vi "Allocate Memory.vi"(4 "Type":variant, 5 "error in (no error)":errorcluster, 8 "Size":i32) -> (0 "Error out":errorcluster, 3 "Data Pointer":i32)   [LabVIEW 2011]
doc: "This VI allocates memory on the heap from LabVIEW and returns a pointer to that memory. If the <B>Type</B> input is wired, then the VI allocates enough memory for <B>Size</B> elements of that type. Otherwise, <B>Size</B> refers to the number of bytes to allocate. Memory allocated by this VI can then be accessed in LabVIEW using the pointer VIs and can also be accessed from other applications or external code. \n\n*Note -This VI allocates memory each time it is run. The operating system will automatically free this memory when the LabVIEW application is closed, not when the VI is complete. To explicitely free memory, use the <B>Free Memory.VI</B>. Failure to do so can result in memory leaks."
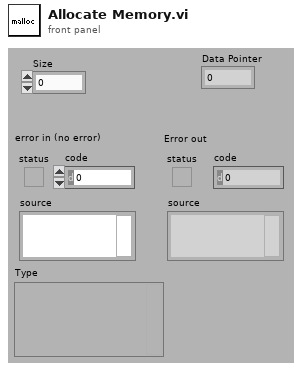
[diagram p1: front panel]
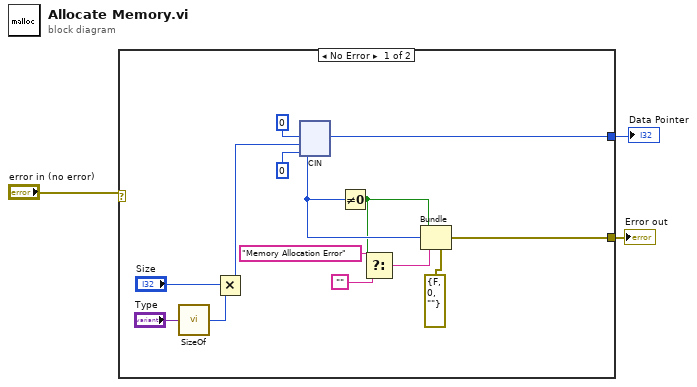
[diagram p0: block diagram]
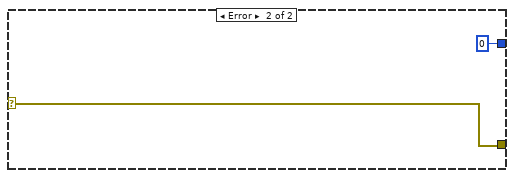
[diagram p2: hidden frame]
diagram:
  n1 = case shown="No Error" "error in (no error)" {
    selector: "error in (no error)" -> [_ w18]
    tunnel: [w16 0] -> w2
    tunnel: [w12 w18] -> w1
    frame No Error {
      n2 = call "SizeOf.vi"("Data"="Type") -> ("Size"=w10:i32)
      n3 = Multiply(x="Size", y=w10) -> (x*y=w8:i32)
      n4 = cin(0, w8, 0) -> (w16:i32, w13:i32)  [unwired: 1 in]
      n5 = Not Equal To 0?(x=w13) -> (x != 0?=w7:bool)
      n6 = Select(t="Memory Allocation Error" ("source"), s=w7, f="") -> (s? t:f=w4:string)
      n7 = Bundle(cluster=errorcluster {"status"=FALSE, "code"=0, "source"=""} ("error IO"), "status"=w7, "code"=w13, "source"=w4) -> (w12:errorcluster)
    }
    frame Error {
    }
  }
  "Data Pointer" <- w2
  "Error out" <- w1
